vi "PID Autotuning Design (Cohen-Coon).vi"(6 "Controller Gain (K)":dbl, 7 "Type of Controller":u16(ring) items=["P", "PI", "PID", "PD"], 8 "dt (s)":dbl, 9 "closed-loop?":bool, 10 "Response signal":dbl[](array[numeric]), 11 "Stimulus signal":dbl[](array[numeric])) -> (1 "PID gains":T2, 2 "response offset":dbl, 3 "stimulus offset":dbl, 4 "Plant Parameters":T1)   [LabVIEW 2017, in "NI_PID_autopid.lvlib"]
doc: "Implements autotuning using the tuning method associated with the polymorphic instance you select. This VI generates PID parameters based on the <B>Stimulus signal</B> and <B>Response signal</B> you specify. You can use this VI to generate initial parameters when you do not have sufficient information about the system you want to tune. You must manually select the polymorphic instance to use."
uses:
  <vilib>/addons/control/pid/NI_PID_autopid.lvlib
  <vilib>/addons/control/pid/pid.llb/PID Structure Conversion (DBL).vi
  <vilib>/addons/control/pid/NI_PID_pid.lvlib
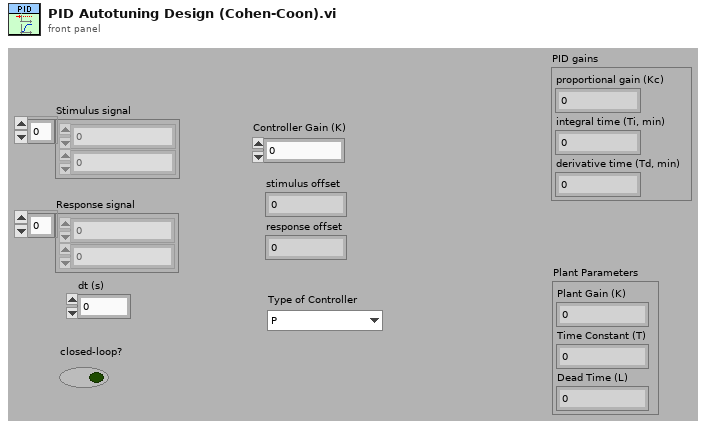
[diagram p1: front panel]
types:
  T1 = cluster{"Plant Gain (K)":dbl, "Time Constant (T)":dbl, "Dead Time (L)":dbl}
  T2 = cluster{"proportional gain (Kc)":dbl, "integral time (Ti, min)":dbl, "derivative time (Td, min)":dbl}
  T3 = enum16{"Academic (Standard)", "Parallel", "Series"}
  T4 = cluster{"OL Gain (Kp)":dbl, "OL Time Constant (T)":dbl, "Dead Time (L) Out":dbl}
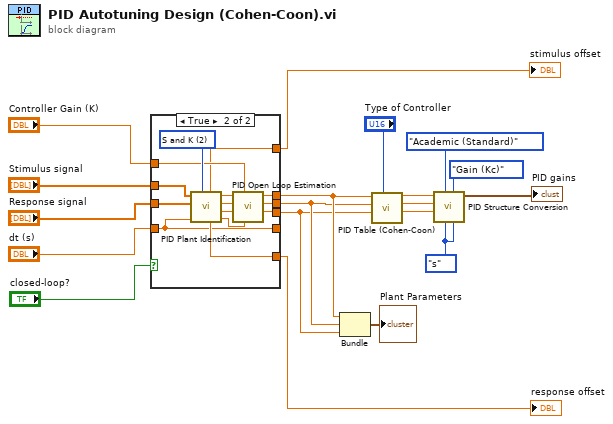
[diagram p0: block diagram]
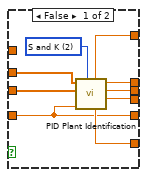
[diagram p2: hidden frame]
diagram:
  w13 = enum16{"min", "s"}."s" ("Integral Unit")
  n1 = case shown="True" "closed-loop?" {
    tunnel: "Response signal" -> [w27 w40]
    tunnel: "Stimulus signal" -> [w26 w41]
    tunnel: [w25 w32] -> w8
    tunnel: [w24 w31] -> w7
    tunnel: [w23 w38] -> w3
    tunnel: [w22 w39] -> w2
    tunnel: [w21 w30] -> w1
    tunnel: "dt (s)" -> [w20 w29]
    tunnel: "Controller Gain (K)" -> [_ w33]
    tunnel: [w20 w29] -> _
    frame False {
      w28 = u16 2 items=["Z-N", "First Order", "S and K"] ("Ring")
      n2 = call <vilib>:"PID Plant Identification.vi"("Method"=w28, "Sampling Time"=w20, "Response signal"=w27, "Stimulus signal"=w26) -> ("Dead Time (L)"=w21:dbl, "Time Constant (T)"=w22:dbl, "Plant Gain (K)"=w23:dbl, "response offset"=w24:dbl, "stimulus offset"=w25:dbl)  [unwired: 1 in, 2 out]
    }
    frame True {
      w42 = u16 2 items=["Z-N", "First Order", "S and K", "Second Order"] ("Method")
      n3 = call <vilib>:"PID Plant Identification.vi"("Method"=w42, "Sampling Time"=w29, "Response signal"=w40, "Stimulus signal"=w41) -> ("Time Constant (T) 2"=w34:dbl, "Dead Time (L)"=w35:dbl, "Time Constant (T)"=w36:dbl, "Plant Gain (K)"=w37:dbl, "response offset"=w31:dbl, "stimulus offset"=w32:dbl)  [unwired: 1 in, 1 out]
      n4 = call <vilib>:"PID Open Loop Estimation.vi"("CL Time Constant (T) 2"=w34, "Controller Gain (K)"=w33, "Dead Time (L)"=w35, "CL Time Constant (Tcl)"=w36, "CL Gain (Kcl)"=w37) -> ("Dead Time (L) Out"=w30:dbl, "OL Time Constant (T)"=w39:dbl, "OL Gain (Kp)"=w38:dbl)  [unwired: 4 in]
    }
  }
  "stimulus offset" <- w8
  "response offset" <- w7
  n5 = Bundle("OL Gain (Kp)"=w3, "OL Time Constant (T)"=w2, "Dead Time (L) Out"=w1) -> (→"Plant Parameters":T4)  [unwired: 1 in]
  n6 = call <vilib>:"PID Table (Cohen-Coon).vi"("Type of Controller"="Type of Controller", "Dead Time (L)"=w1, "Time Constant (T)"=w2, "Plant Gain (K)"=w3) -> ("Derivative Time (Td)"=w16:dbl, "Integral Time (Ti)"=w17:dbl, "Proportional Gain (Kp)"=w18:dbl)  [unwired: 5 in]
  n7 = call-poly <vilib>:"PID Structure Conversion.vi"("derivative unit"=w13, "proportional unit"=enum16{"Gain (Kc)", "Band (PB)"}."Gain (Kc)" ("Proportional Unit"), "integral unit"=w13, "PID structure"=T3."Academic (Standard)" ("PID Structure"), "derivative"=w16, "integral"=w17, "proportional"=w18) -> ("PID gains"=→"PID gains":T2)  [unwired: 4 in]
